vi "Hold.vi"(8 "error in (no error)":errorcluster, 11 "Instrument.1820 in":refnum<class "Instrument.Oxford1820.lvclass">) -> (0 "error out":errorcluster, 2 "Response":string, 3 "Instrument.1820 in":refnum<class "Instrument.Oxford1820.lvclass">)   [LabVIEW 2019, in "Instrument.Oxford1820.lvclass"]
uses:
  Instrument.Oxford1820.lvclass
  C:/Program Files (x86)/National Instruments/LabVIEW 2019/user.lib/LevyLab/Instrument Framework/SMOs/Instrument/Instrument.lvclass
  <instrlib>/Mercury iXX/Public/Libraries/Magnet/Controls/PSU Actions.ctl
  Typedefs/Instrument.Oxford1820.publicCommands-enum.ctl
  <userlib>/LevyLab/Instrument Framework/SMOs/Instrument/Instrument.lvclass/Instrument.ctl
  548c5cec-5e13-40ab-b4cc-26b923086f95.vi
  548c5cec-5e13-40ab-b4cc-26b923086f95.vi/b0c5fdac-0c3f-4d27-9cb1-80da4ad29970.vi
  548c5cec-5e13-40ab-b4cc-26b923086f95.vi/d6affe4c-f68c-4c89-a836-5fc9f7ea2699.vi
  548c5cec-5e13-40ab-b4cc-26b923086f95.vi/b0c5fdac-0c3f-4d27-9cb1-80da4ad29970.vi/092a7611-668f-471c-9638-24e4c7571422.vi
  <userlib>/LevyLab/Instrument Framework/SMOs/Instrument/API/Send and Receive.vi
  548c5cec-5e13-40ab-b4cc-26b923086f95.vi/b0c5fdac-0c3f-4d27-9cb1-80da4ad29970.vi/084e782e-bf95-48f6-a5e7-151391d3f8cf.vi
  <userlib>/LevyLab/Instrument Framework/SMOs/Instrument/Private/Get Client Type.vi
  548c5cec-5e13-40ab-b4cc-26b923086f95.vi/d6affe4c-f68c-4c89-a836-5fc9f7ea2699.vi/99c05e22-f0dd-4008-9ecf-6ede6bc4f0ea.vi
  548c5cec-5e13-40ab-b4cc-26b923086f95.vi/d6affe4c-f68c-4c89-a836-5fc9f7ea2699.vi/9a3944fd-5260-42dc-9e72-668670251da1.vi
  548c5cec-5e13-40ab-b4cc-26b923086f95.vi/b0c5fdac-0c3f-4d27-9cb1-80da4ad29970.vi/092a7611-668f-471c-9638-24e4c7571422.vi/4339722b-900c-4e43-842e-290fe32090bf.vi
  548c5cec-5e13-40ab-b4cc-26b923086f95.vi/b0c5fdac-0c3f-4d27-9cb1-80da4ad29970.vi/092a7611-668f-471c-9638-24e4c7571422.vi/a8e355f0-b6d6-4534-9de5-f06d9dda8930.vi
  548c5cec-5e13-40ab-b4cc-26b923086f95.vi/b0c5fdac-0c3f-4d27-9cb1-80da4ad29970.vi/084e782e-bf95-48f6-a5e7-151391d3f8cf.vi/a2c3ddd2-211b-4dab-be4e-d90c0ff2d315.vi
  548c5cec-5e13-40ab-b4cc-26b923086f95.vi/b0c5fdac-0c3f-4d27-9cb1-80da4ad29970.vi/084e782e-bf95-48f6-a5e7-151391d3f8cf.vi/4e6e9645-73d6-4511-87b8-f9bf59523b1a.vi
  548c5cec-5e13-40ab-b4cc-26b923086f95.vi/b0c5fdac-0c3f-4d27-9cb1-80da4ad29970.vi/084e782e-bf95-48f6-a5e7-151391d3f8cf.vi/a2c3ddd2-211b-4dab-be4e-d90c0ff2d315.vi/5130f0d1-30a7-4076-8597-908e6d05eb52.vi
  548c5cec-5e13-40ab-b4cc-26b923086f95.vi/b0c5fdac-0c3f-4d27-9cb1-80da4ad29970.vi/084e782e-bf95-48f6-a5e7-151391d3f8cf.vi/a2c3ddd2-211b-4dab-be4e-d90c0ff2d315.vi/ae944916-c794-4b72-8ac7-ed7b57370bcf.vi
  <userlib>/LevyLab/Instrument Framework/SMOs/Instrument/Private/Get RC Connection Status.vi
  <userlib>/LevyLab/Instrument Framework/SMOs/Instrument/API/Enum to String.vi
  <userlib>/LevyLab/Instrument Framework/SMOs/RemoteControl/API/Send and Receive.vi
  <vilib>/Utility/Data Type/Get Type Information.vi
  <vilib>/JDP Science/JSONtext/JSON text to Variant.vi
  <userlib>/LevyLab/Instrument Framework/SMOs/Instrument/API/Instrument.GetPublicEvents.vi
  <vilib>/JDP Science/JSONtext/Variant to JSON Text.vi
  <vilib>/National Instruments/GUID Generator/Guid Generator.vi
  <userlib>/LevyLab/Instrument Framework/SMOs/Instrument/API/Instrument.MessageToProcess.vi
  <userlib>/LevyLab/Instrument Framework/SMOs/Instrument/Private/Instrument.MessageFromProcess.EventStructure.vi
  <vilib>/JDP Science/JSONtext/LVClass Serializer/JSONtext LVClass Serializer.lvclass
  <instrlib>/Mercury iXX/Public/Libraries/Magnet.lvlib
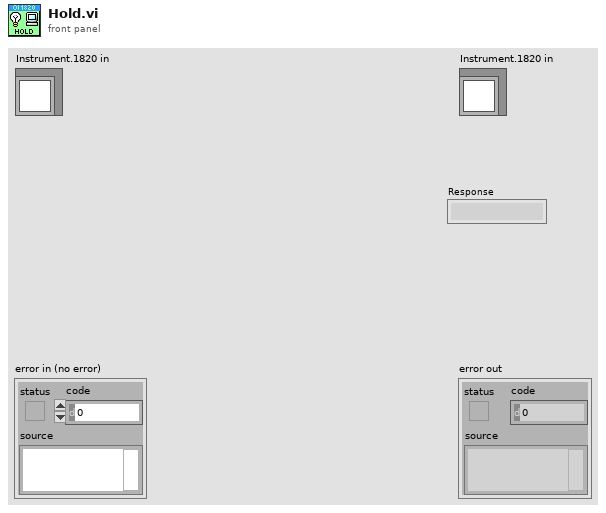
[diagram p1: front panel]
types:
  T1 = typedef "Instrument.Oxford1820.lvclass/Instrument.Oxford1820.publicCommands-enum.ctl" = enum16{"setMagnetField", "getMagnetField"}
  T2 = typedef "Mercury iXX.lvlib/Magnet.lvlib/PSU Actions.ctl" = string
  T3 = cluster{"Holding":bool, "Ramp to Setpoint":bool, "Ramp to Zero":bool, "Clamp":bool}
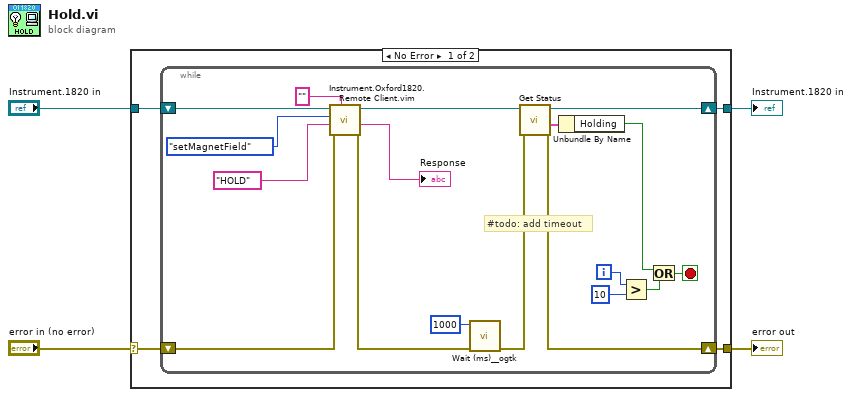
[diagram p0: block diagram]
diagram:
  n1 = case shown="No Error" "error in (no error)" {
    selector: "error in (no error)" -> [w7 w28]
    tunnel: [w5 w28] -> w3
    tunnel: [w6 w27] -> w1
    tunnel: "Instrument.1820 in" -> [w8 w27]
    frame No Error {
      n2 = while {
        shift-right: [w18] -> w6
        shift-left: w8 -> [w19]
        shift-right: [w23] -> w5
        shift-left: w7 -> [w24]
        i -> [w13]
        stop <- w15 stop-if-true
        # "#todo: add timeout"
        n3 = call "Instrument.Oxford1820.Remote Client.vim"("Data Out type"="", "error in (no error)"=w24, "Data"=T2 "HOLD" ("PSU Act Stat"), "Commands"=Instrument.Oxford1820.publicCommands-enum."setMagnetField", "Instrument.1820 in"=w19) -> ("error out"=w12:errorcluster, "Data out"=→"Response":string, "Instrument.1820 out"=w11:refnum<class "Instrument.Oxford1820.lvclass">)  [unwired: 4 in]
        n4 = call <userlib>:"Wait (ms)__ogtk.vi"("error in (no error)"=w12, "milliseconds to wait"=u32 1000) -> ("error out"=w22:errorcluster)  [unwired: 8 in, 1 out]
        n5 = call "Get Status.vi"("error in (no error)"=w22, "Instrument.1820 in"=w11) -> ("error out"=w23:errorcluster, "Status"=w20:T3, "Instrument.1820 in"=w18:refnum<class "Instrument.Oxford1820.lvclass">)  [unwired: 6 in, 1 out]
        n6 = Unbundle By Name(w20) -> ("Holding"=w14:bool)
        n7 = Greater?(x=w13, y=10) -> (0:w16:bool)
        n8 = Or(x=w14, y=w16) -> (x .or. y?=w15:bool)
      }
    }
    frame Error {
    }
  }
  "error out" <- w3
  "Instrument.1820 in" <- w1
